vi "Yokogawa WT300 Series Reset Integrator.vi"(7 "Initialization Routing?":bool, 8 "Error In":errorcluster, 11 "VISA Refnum in":refnum<visa-resource-name>) -> (0 "Error Out":errorcluster, 3 "VISA resource name out":refnum<visa-resource-name>)   [LabVIEW 2019]
uses:
  Yokogawa WT300 Series.lvlib
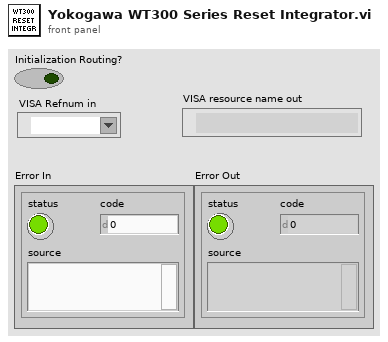
[diagram p1: front panel]
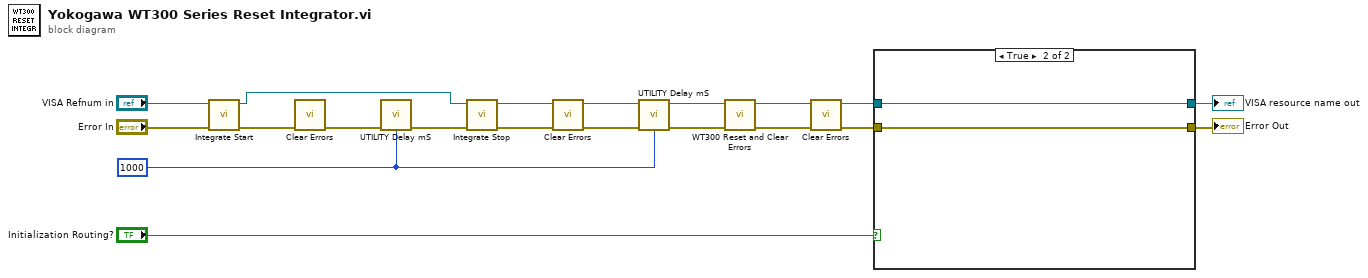
[diagram p0: block diagram]
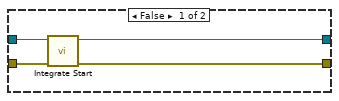
[diagram p2: hidden frame]
diagram:
  w7 = u32 1000 ("milliseconds to wait")
  n1 = call "Integrate Start.vi"("error in (no error)"="Error In", "VISA resource name"="VISA Refnum in") -> ("error out"=w13:errorcluster, "VISA resource name out"=w10:refnum<visa-resource-name>)  [unwired: 8 in]
  n2 = call <vilib>:"Clear Errors.vi"("error in (no error)"=w13) -> ("error out"=w14:errorcluster)  [unwired: 5 in, 1 out]
  n3 = call "UTILITY Delay mS.vi"("Error In"=w14, "milliseconds to wait"=w7) -> ("Error Out"=w11:errorcluster)  [unwired: 13 in]
  n4 = call "Integrate Stop.vi"("error in (no error)"=w11, "VISA resource name"=w10) -> ("error out"=w15:errorcluster, "VISA resource name out"=w9:refnum<visa-resource-name>)  [unwired: 8 in]
  n5 = call <vilib>:"Clear Errors.vi"("error in (no error)"=w15) -> ("error out"=w16:errorcluster)  [unwired: 5 in, 1 out]
  n6 = call "UTILITY Delay mS.vi"("Error In"=w16, "milliseconds to wait"=w7) -> ("Error Out"=w8:errorcluster)  [unwired: 13 in]
  n7 = call "WT300 Reset and Clear Errors.vi"("error in (no error)"=w8, "VISA Refnum in"=w9) -> ("error out"=w1:errorcluster, "VISA Refnum out"=w2:refnum<visa-resource-name>)  [unwired: 8 in]
  n8 = call <vilib>:"Clear Errors.vi"("error in (no error)"=w1) -> ("error out"=w17:errorcluster)  [unwired: 5 in, 1 out]
  n9 = case shown="True" "Initialization Routing?" {
    tunnel: w17 -> [w21 w22]
    tunnel: w2 -> [w20 w23]
    tunnel: [w19 w22] -> w4
    tunnel: [w18 w23] -> w3
    frame False {
      n10 = call "Integrate Start.vi"("error in (no error)"=w21, "VISA resource name"=w20) -> ("error out"=w19:errorcluster, "VISA resource name out"=w18:refnum<visa-resource-name>)  [unwired: 8 in]
    }
    frame True {
    }
  }
  "Error Out" <- w4
  "VISA resource name out" <- w3
